vi "OnResize2.vi"(0 "XRef":T10, 1 "Bounds":T9, 2 "Mouse Mods":T7, 3 "State In":T1) -> (14 "Reply":T5, 15 "Fatal Error Out":T4, 16 "State Out":T1)   [LabVIEW 2021, in "FirstXNode .xnode"]
uses:
  FirstXNode .xnode
  <vilib>/XNodeSupport/XNodeXNodeRef.ctl
  <vilib>/XNodeSupport/XNodeRect32.ctl
  <vilib>/XNodeSupport/XNodeInt.ctl
  <vilib>/XNodeSupport/XNodeMouseMods.ctl
  <vilib>/XNodeSupport/XNodeBool.ctl
  State.ctl
  <vilib>/XNodeSupport/XNodeBounds.ctl
  <vilib>/XNodeSupport/XNodeStringArray.ctl
  <vilib>/XNodeSupport/XNodeString.ctl
  <vilib>/XNodeSupport/XNodeErrorCluster.ctl
  <vilib>/XNodeSupport/NI_XNodeSupport.lvlib
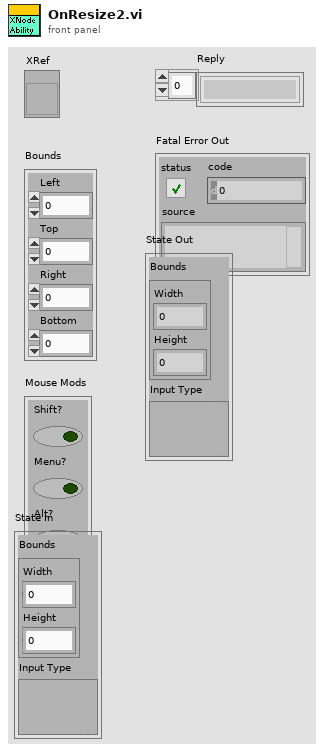
[diagram p1: front panel]
types:
  T1 = typedef "FirstXNode .xnode/State.ctl" = cluster{"Bounds":T2, "Input Type":variant}
  T2 = typedef "NI_XNodeSupport.lvlib/XNodeBounds.ctl" = cluster{"Width":T3, "Height":T3}
  T3 = typedef "NI_XNodeSupport.lvlib/XNodeInt.ctl" = i32
  T4 = typedef "NI_XNodeSupport.lvlib/XNodeErrorCluster.ctl" = errorcluster
  T5 = typedef "NI_XNodeSupport.lvlib/XNodeStringArray.ctl" = T6[]
  T6 = typedef "NI_XNodeSupport.lvlib/XNodeString.ctl" = string
  T7 = typedef "NI_XNodeSupport.lvlib/XNodeMouseMods.ctl" = cluster{"Shift?":T8, "Menu?":T8, "Alt?":T8}
  T8 = typedef "NI_XNodeSupport.lvlib/XNodeBool.ctl" = bool
  T9 = typedef "NI_XNodeSupport.lvlib/XNodeRect32.ctl" = cluster{"Left":T3, "Top":T3, "Right":T3, "Bottom":T3}
  T10 = typedef "NI_XNodeSupport.lvlib/XNodeXNodeRef.ctl" = refnum<vi>
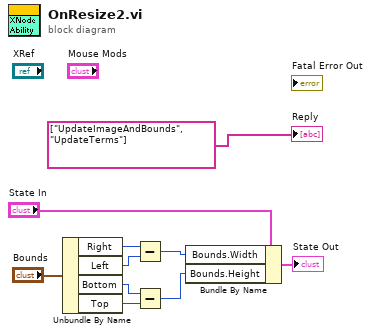
[diagram p0: block diagram]
diagram:
  n1 = Unbundle By Name("Bounds") -> ("Right"=w6:T3, "Left"=w5:T3, "Bottom"=w4:T3, "Top"=w3:T3)
  n2 = Subtract(x=w6, y=w5) -> (x-y=w7:T3)
  n3 = Subtract(x=w4, y=w3) -> (x-y=w8:T3)
  n4 = Bundle By Name(cluster="State In", "Bounds.Width"=w7, "Bounds.Height"=w8) -> (→"State Out":T1)
  "Reply" <- T5 ["UpdateImageAndBounds", "UpdateTerms"] ("Reply")
